vi "Mesure_nyquist_parametrise.vi"() -> ()   [LabVIEW 2013]
uses:
  <vilib>/gmath/NI_Gmath.lvlib
  <vilib>/Analysis/NI_AALPro.lvlib
panel:
  out "Signal interpolé fourier":dbl[](graph)
  out "Signal interpolé polynomial":i32[](graph)
  in  "Nombre de données de sortie":dbl
  out "Signal mesuré":dynamicdata(graph)
  out "Nombre d'échantillons":dbl
  in  "Fréquence d'échantillonnage":dbl
  in  "Fréquence du signal":dbl
  in  "Nombre de cycles":dbl
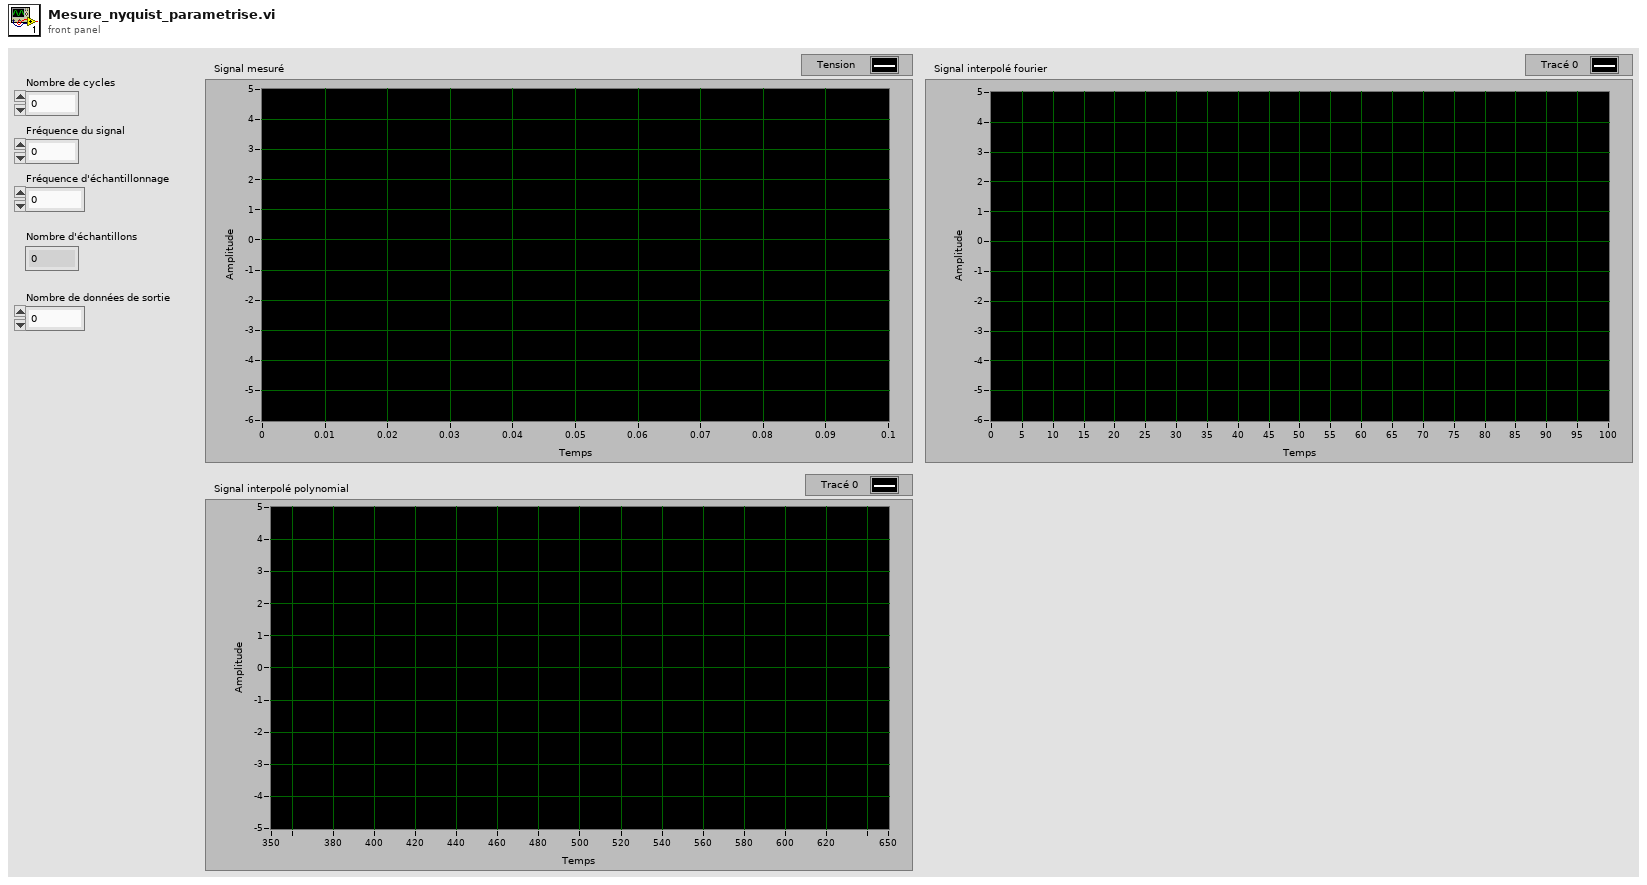
[diagram p1: front panel]
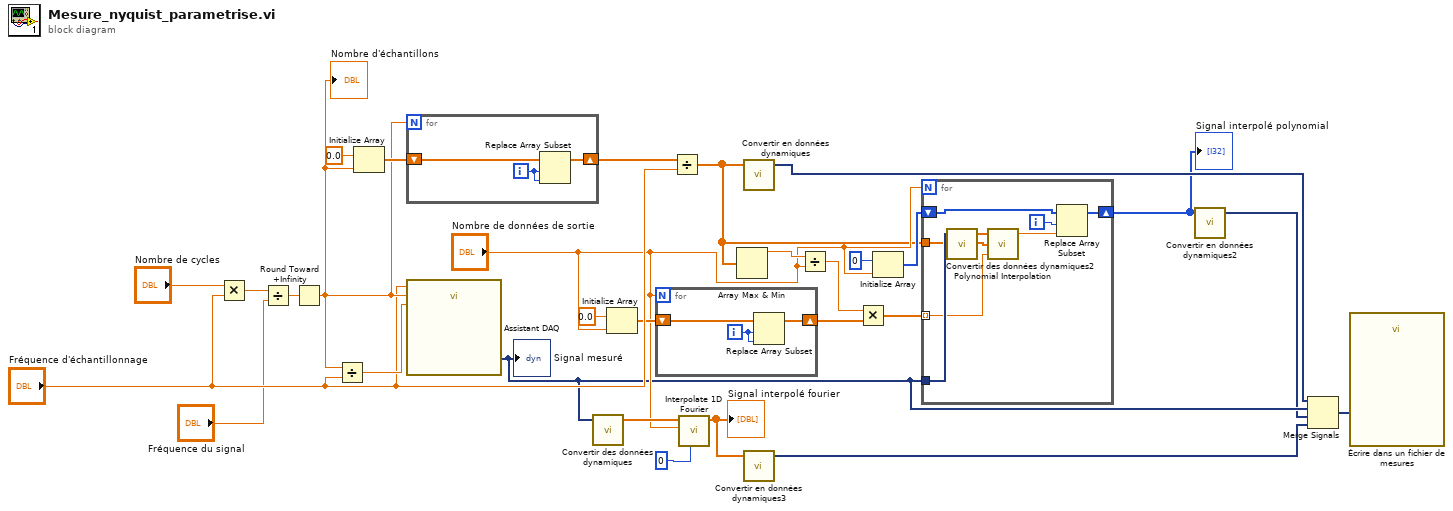
[diagram p0: block diagram]
diagram:
  n1 = Multiply(x="Nombre de cycles", y="Fréquence d'échantillonnage") -> (x*y=w29:dbl)
  n2 = Divide(x=w29, y="Fréquence du signal") -> (x/y=w28:dbl)
  n3 = Round Toward +Infinity(x=w28) -> (ceil(x): smallest int >= x=w22:dbl)
  "Nombre d'échantillons" <- w22
  n4 = Divide(x=w22, y="Fréquence d'échantillonnage") -> (x/y=w27:dbl)
  n5 = Initialize Array(0.0, w22) -> (w26:dbl[])
  n6 = for {
    N: w22 -> [_]
    shift-right: [w31] -> w9
    shift-left: w26 -> [w30]
    i -> [w32]
    n7 = Replace Array Subset(array=w30, new element=w32, index=w32) -> (w31:dbl[])
  }
  n8 = call "Assistant DAQ"("vitesse"="Fréquence d'échantillonnage", "nombre d'échantillons"=w22, "timeout (s)"=w27) -> ("data"=w5:dynamicdata)  [unwired: 14 in, 2 out]
  "Signal mesuré" <- w5
  n9 = call "Convertir des données dynamiques"("Dynamic Data Type"=w5) -> ("Array"=w13:dbl[])  [unwired: 3 in]
  n10 = Initialize Array(0.0, "Nombre de données de sortie") -> (w19:dbl[])
  n11 = for {
    N: "Nombre de données de sortie" -> [_]
    shift-right: [w34] -> w15
    shift-left: w19 -> [w33]
    i -> [w35]
    n12 = Replace Array Subset(array=w33, new element=w35, index=w35) -> (w34:dbl[])
  }
  n13 = Divide(x=w9, y="Fréquence d'échantillonnage") -> (x/y=w7:dbl[])
  n14 = call <vilib>:"Interpolate 1D Fourier.vi"("type"=0, "n"="Nombre de données de sortie", "X"=w13) -> ("Y"=w2:dbl[])  [unwired: 5 in, 3 out]
  "Signal interpolé fourier" <- w2
  n15 = Array Max & Min(array=w7) -> (max value=w17:dbl)  [unwired: 3 out]
  n16 = call "Convertir en données dynamiques"("Array"=w7) -> ("Dynamic Data Type"=w23:dynamicdata)  [unwired: 3 in]
  n17 = call "Convertir en données dynamiques3"("Array"=w2) -> ("Dynamic Data Type"=w1:dynamicdata)  [unwired: 3 in]
  n18 = Divide(x=w17, y="Nombre de données de sortie") -> (x/y=w16:dbl)
  n19 = Multiply(x=w16, y=w15) -> (x*y=w6:dbl[])
  n20 = Initialize Array(0, "Nombre de données de sortie") -> (w10:i32[])
  n21 = for {
    N: "Nombre de données de sortie" -> [_]
    shift-right: [w40] -> w4
    shift-left: w10 -> [w41]
    tunnel: w5 -> [w39]
    tunnel: w7 -> [w37]
    tunnel: w6 -> [w36] mode=indexing
    i -> [w42]
    n22 = call "Convertir des données dynamiques2"("Dynamic Data Type"=w39) -> ("Array"=w38:dbl[])  [unwired: 3 in]
    n23 = call <vilib>:"Polynomial Interpolation.vi"("x value"=w36, "X"=w37, "Y"=w38) -> ("interpolation value"=w43:dbl)  [unwired: 2 out]
    n24 = Replace Array Subset(array=w41, new element=w43, index=w42) -> (w40:i32[])
  }
  "Signal interpolé polynomial" <- w4
  n25 = call "Convertir en données dynamiques2"("Array"=w4) -> ("Dynamic Data Type"=w3:dynamicdata)  [unwired: 3 in]
  n26 = Merge Signals ("Assembler des signaux")(w23, w5, w3, w1) -> (w24:dynamicdata)
  n27 = call "Écrire dans un fichier de mesures"("Signals"=w24) -> ()  [unwired: 16 in, 3 out]
